vi "Check Action.vi"(6 "HRS Time":dbl, 7 "Values In":dbl[](array[numeric]), 8 "error in (no error)":errorcluster, 11 "SequencedValves in":refnum<class "SequencedValves.lvclass">) -> (0 "error out":errorcluster, 1 "Do Action":bool, 2 "Action":T1, 3 "SequencedValves out":refnum<class "SequencedValves.lvclass">, 5 "Values":dbl[](array[numeric]))   [LabVIEW 2020, in "VolatusControl.lvlib" / "SequencedValves.lvclass"]
uses:
  SequencedValves.lvclass
  Valve Action.ctl
  Volatus/MessageQ/MessageQ.lvclass
  SequencedValves.lvclass/SequencedValves.ctl
  State.ctl
  VolatusControl.lvlib
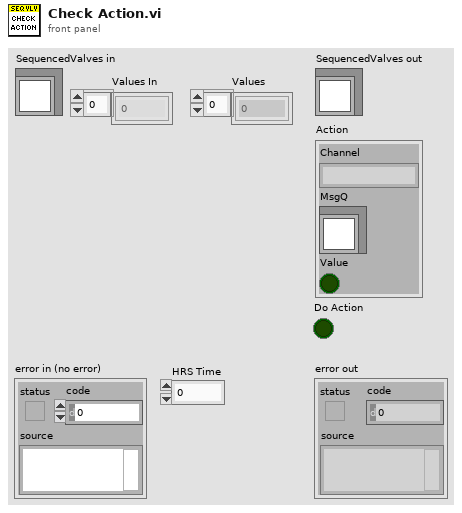
[diagram p1: front panel]
types:
  T1 = typedef "VolatusControl.lvlib/Valve Action.ctl" = cluster{"Channel":string, "MsgQ":refnum<class "MessageQ.lvclass">, "Value":bool}
  T2 = typedef "VolatusControl.lvlib/SequencedValves.lvclass/State.ctl" = enum16{"Idle", "Start", "Delay"}
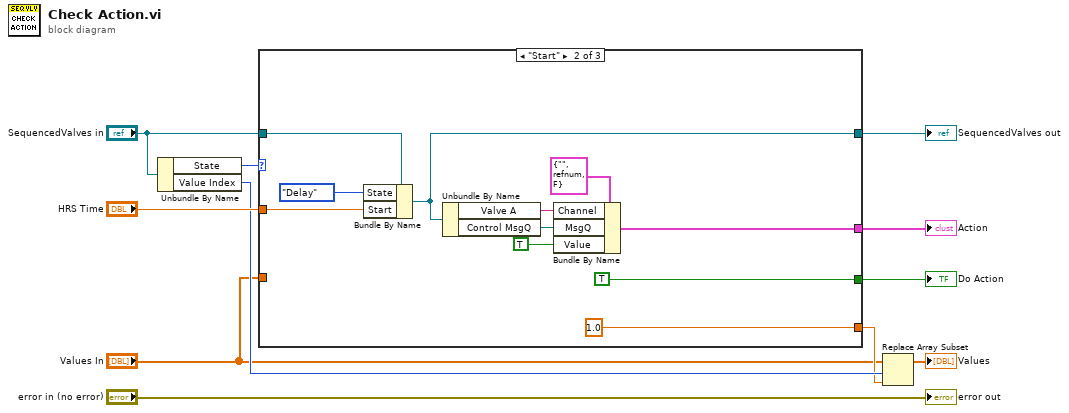
[diagram p0: block diagram]
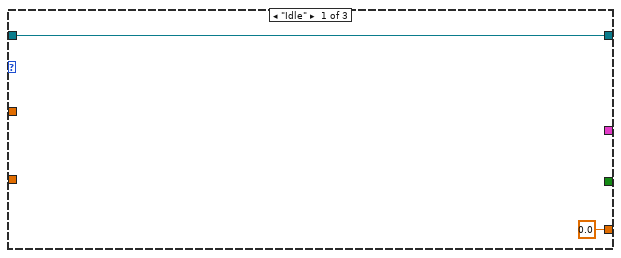
[diagram p2: hidden frame]
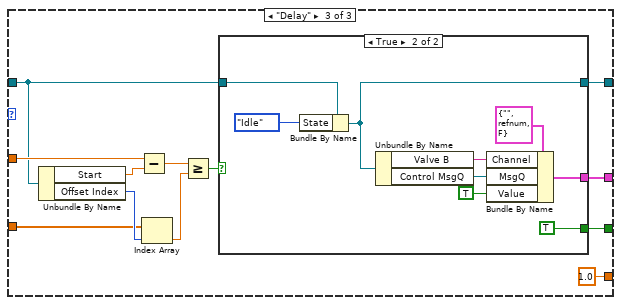
[diagram p3: hidden frame]
diagram:
  n1 = Unbundle By Name("SequencedValves in") -> ("State"=w10:T2, "Value Index"=w3:i32)
  n2 = case shown="\"Start\"" w10 {
    tunnel: "SequencedValves in" -> [w13 w21 w32]
    tunnel: "HRS Time" -> [_ w19 w36]
    tunnel: [w13 w18 w31] -> w7
    tunnel: [_ w23 w30] -> w6
    tunnel: [_ TRUE w29] -> w5
    tunnel: [0.0 1.0 1.0] -> w2
    tunnel: "Values In" -> [_ _ w27]
    frame "Idle" {
    }
    frame "Start" {
      n3 = Bundle By Name(cluster=w21, "State"=State."Delay", "Start"=w19) -> (w18:refnum<class "SequencedValves.lvclass">)
      n4 = Unbundle By Name(w18) -> ("Valve A"=w16:string, "Control MsgQ"=w17:refnum<class "MessageQ.lvclass">)
      n5 = Bundle By Name(cluster=T1 {"Channel"="", "MsgQ"=refnum, "Value"=FALSE} ("Action"), "Channel"=w16, "MsgQ"=w17, "Value"=TRUE) -> (w23:T1)
    }
    frame "Delay" {
      n6 = Unbundle By Name(w32) -> ("Start"=w35:dbl, "Offset Index"=w28:i32)
      n7 = Subtract(x=w36, y=w35) -> (x-y=w34:dbl)
      n8 = Index Array(array=w27, index=w28) -> (element=w26:dbl)
      n9 = Greater Or Equal?(x=w34, y=w26) -> (x >= y?=w33:bool)
      n10 = case shown="True" w33 {
        tunnel: w32 -> [w37 w40]
        tunnel: [w37 w39] -> w31
        tunnel: [_ w42] -> w30
        tunnel: [_ TRUE] -> w29
        frame False {
        }
        frame True {
          n11 = Bundle By Name(cluster=w40, "State"=State."Idle") -> (w39:refnum<class "SequencedValves.lvclass">)
          n12 = Unbundle By Name(w39) -> ("Valve B"=w43:string, "Control MsgQ"=w44:refnum<class "MessageQ.lvclass">)
          n13 = Bundle By Name(cluster=T1 {"Channel"="", "MsgQ"=refnum, "Value"=FALSE} ("Action"), "Channel"=w43, "MsgQ"=w44, "Value"=TRUE) -> (w42:T1)
        }
      }
    }
  }
  "SequencedValves out" <- w7
  "Action" <- w6
  "Do Action" <- w5
  n14 = Replace Array Subset(array="Values In", new element=w2, index=w3) -> (→"Values":dbl[])
  "error out" <- "error in (no error)"
